vi "Launcher.vi"() -> ()   [LabVIEW 2020]
uses:
  [P] User/[P] User/[P] User.lvclass
  C:/Program Files (x86)/National Instruments/LabVIEW 2020/vi.lib/ActorFramework/Actor/Actor.lvclass
  [P] User/[P] User/[P] User.lvclass/[P] User.ctl
  <vilib>/ActorFramework/Message Enqueuer/Message Enqueuer.lvclass/Message Enqueuer.ctl
  <vilib>/ActorFramework/Message/Message.lvclass
  [P] User/[P] User/Accessor/Write Software Name.vi
  [P] User/[P] User/Accessor/Write Recent User File.vi
  [P] User/[P] User/Accessor/Write Userinfo File.vi
  [P] User/[P] User/Accessor/Write Config File.vi
  <vilib>/ActorFramework/Stop Msg/Stop Msg.lvclass
  C:/Program Files (x86)/National Instruments/LabVIEW 2020/vi.lib/ActorFramework/Message/Message.lvclass
  <vilib>/ActorFramework/Message Priority Queue/Priority Enqueue.vi
  <vilib>/ActorFramework/Actor/Actor.lvclass
  <vilib>/ActorFramework/Message Enqueuer/Message Enqueuer.lvclass
panel:
  in  "self info":bool
  in  "user list":bool
  # "Launcher"
  # "超级管理员 用户名：root\n管理员       用户名：admin\n操作员       用户名：operator"
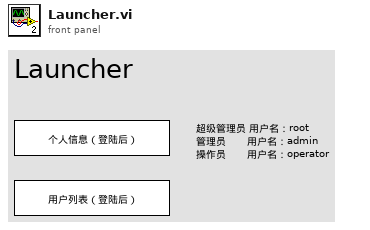
[diagram p1: front panel]
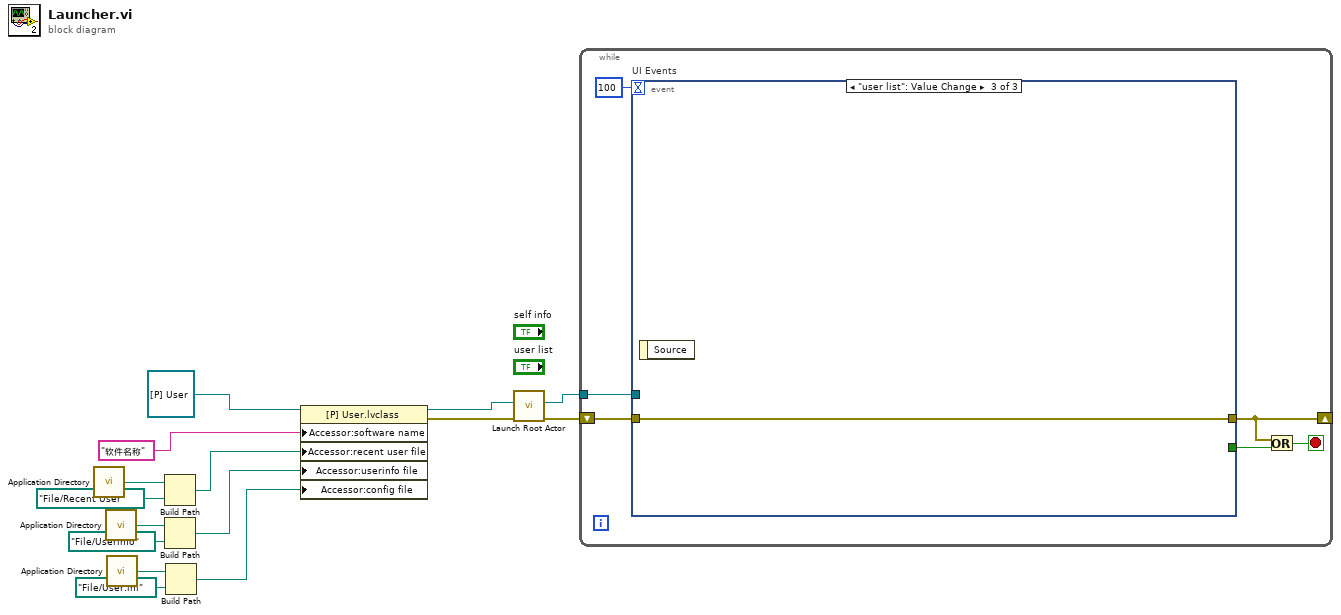
[diagram p0: block diagram]
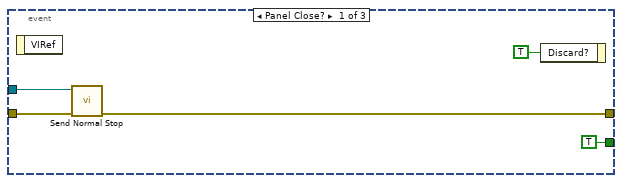
[diagram p2: hidden frame]
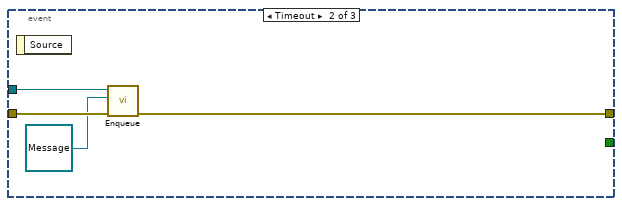
[diagram p3: hidden frame]
diagram:
  n1 = call <vilib>:"Application Directory.vi"() -> ("Application Directory"=w14:path)
  n2 = call <vilib>:"Application Directory.vi"() -> ("Application Directory"=w9:path)
  n3 = call <vilib>:"Application Directory.vi"() -> ("Application Directory"=w3:path)
  n4 = Build Path(base path=w14, name or relative path=path "File/Recent User") -> (appended path=w13:path)
  n5 = Build Path(base path=w9, name or relative path=path "File/Userinfo") -> (appended path=w5:path)
  n6 = Build Path(base path=w3, name or relative path=path "File/User.ini") -> (appended path=w2:path)
  n7 = property class="[P] User.lvclass"(reference=refnum<class "[P] User.lvclass"> refnum ("[P] User.lvlib:[P] User.lvclass"), "Accessor:software name"="软件名称" ("software name"), "Accessor:recent user file"=w13, "Accessor:userinfo file"=w5, "Accessor:config file"=w2) -> (reference out=w10:refnum<class "[P] User.lvclass">, error out=w11:errorcluster)  [unwired: 1 in]
  n8 = call <vilib>:"Launch Root Actor.vi"("error in (no error)"=w11, "Actor"=w10) -> ("error out"=w7:errorcluster, "Actor's Enqueuer"=w6:refnum<class "Message Enqueuer.lvclass">)  [unwired: 8 in]
  n9 = while {
    shift-right: [w16] -> _
    shift-left: w7 -> [w21]
    tunnel: w6 -> [w20]
    stop <- w17 stop-if-true
    n10 = event "UI Events" shown="[2] \"user list\": Value Change" {
      selector: _ -> [_ _ _]
      dyn-events: _ -> [_ _ _]
      timeout: 100 -> [_ _ _]
      tunnel: [TRUE ("stop") _ _] -> w18
      tunnel: w21 -> [w24 w30 w31]
      tunnel: [w22 w27 w31] -> w16
      tunnel: w20 -> [w23 w29 _]
      event Panel Close? {
        n11 = event-data() -> ()  [unwired: 1 in, 1 out]
        n12 = call <vilib>:"Send Normal Stop.vi"("error in (no error)"=w24, "Message Enqueuer"=w23) -> ("error out"=w22:errorcluster)  [unwired: 9 in]
        n13 = event-data("Discard?"=TRUE) -> ()  [unwired: 1 in, 1 out]
      }
      event Timeout {
        n14 = event-data() -> ()  [unwired: 1 in, 1 out]
        n15 = call <vilib>:"Enqueue.vi"("error in (no error)"=w30, "Message"=refnum<class "Message.lvclass"> refnum, "Message Enqueuer in"=w29) -> ("error out"=w27:errorcluster)  [unwired: 7 in, 1 out]
      }
      event "user list": Value Change {
        n16 = event-data() -> ()  [unwired: 1 in, 1 out]
      }
    }
    n17 = Or(x=w16, y=w18) -> (x .or. y?=w17:bool)
  }
